vi "Write Return Message Msg.vi"(8 "error in (no error)":errorcluster, 10 "Network Stream.lvlib:Network Stream Return Message Msg.lvclass":refnum<class "Return undeliverable Msg.lvclass">, 11 "Network Stream in":refnum<class "Network Stream.lvclass">) -> (0 "error out":errorcluster, 3 "Network Stream out":refnum<class "Network Stream.lvclass">)   [LabVIEW 2014]
uses:
  Network Stream.lvclass
  Proxy/Proxy Messages/Return undeliverable Msg/Return undeliverable Msg.lvclass
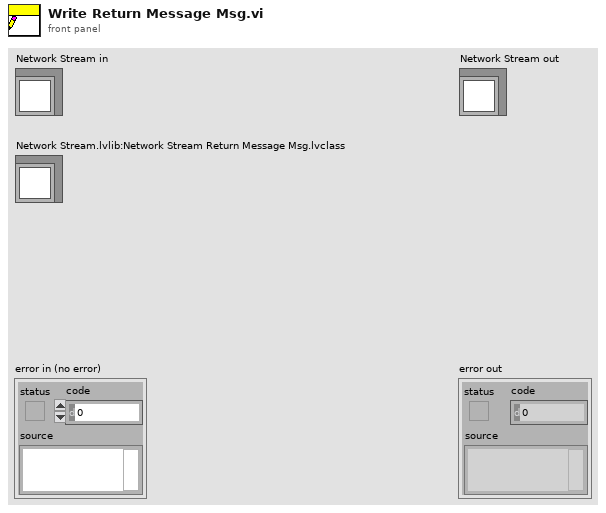
[diagram p1: front panel]
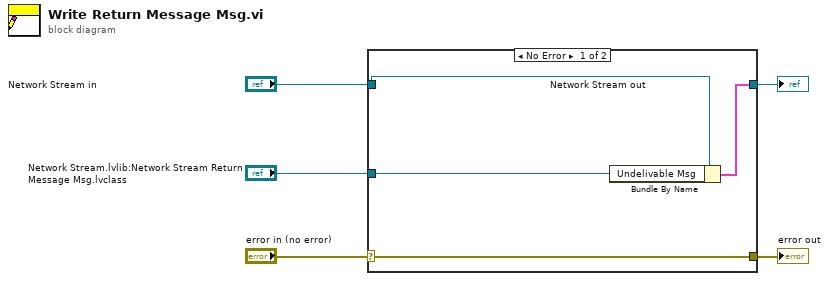
[diagram p0: block diagram]
diagram:
  n1 = case shown="No Error" "error in (no error)" {
    selector: "error in (no error)" -> [w9 w10]
    tunnel: [w9 w10] -> w4
    tunnel: [w7 w11] -> w2
    tunnel: "Network Stream in" -> [w8 w11]
    tunnel: "Network Stream.lvlib:Network Stream Return Message Msg.lvclass" -> [w6 _]
    frame No Error {
      n2 = Bundle By Name(cluster=w8, "Undelivable Msg"=w6) -> (w7:cluster{})
    }
    frame Error {
    }
  }
  "error out" <- w4
  "Network Stream out" <- w2
